vi "Build_Asylum_WriteString.vi"(8 "error in (no error)":errorcluster, 10 "valueString":string, 11 "parameterName":string) -> (0 "error out":errorcluster, 3 "String":string)   [LabVIEW 2019]
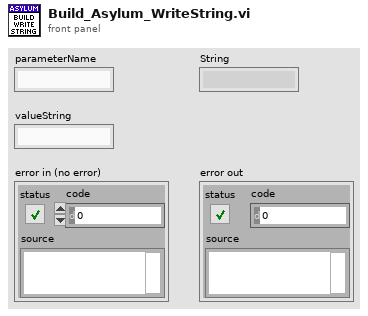
[diagram p1: front panel]
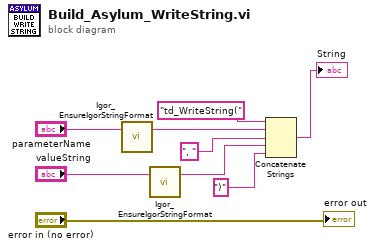
[diagram p0: block diagram]
diagram:
  n1 = call "Igor_EnsureIgorStringFormat.vi"("Value"="parameterName") -> ("Value"=w6:string)  [unwired: 2 in]
  n2 = call "Igor_EnsureIgorStringFormat.vi"("Value"="valueString") -> ("Value"=w9:string)  [unwired: 2 in]
  n3 = Concatenate Strings("td_WriteString(", w6, ", ", w9, ")" ("string")) -> (→"String":string)
  "error out" <- "error in (no error)"
